vi "Saving to Disk.vi"() -> ()   [LabVIEW 2011]
uses:
  <vilib>/Heliosphere Research LLC/Advanced Plotting Toolkit/Advanced Plotting Toolkit.lvlib
  <vilib>/Utility/sysdir.llb/System Directory Type.ctl
  <vilib>/Heliosphere Research LLC/Advanced Plotting Toolkit/properties/Line_Style.ctl
  <vilib>/Heliosphere Research LLC/Advanced Plotting Toolkit/typedefs/PlotColor.ctl
  <vilib>/Heliosphere Research LLC/Advanced Plotting Toolkit/properties/Line.ctl
  <vilib>/Heliosphere Research LLC/Advanced Plotting Toolkit/properties/Display.ctl
  <vilib>/Heliosphere Research LLC/Advanced Plotting Toolkit/api_plotting/ContourProperties.ctl
  <vilib>/Heliosphere Research LLC/Advanced Plotting Toolkit/api_plotting/Contour_Automatic.vi
panel:
  out "Error from Save":errorcluster
  in  "File Name (on your Desktop)":string="SavedPlot.pdf"
  out "Contour Plot":picture
  # "Saving to Disk"
  # "This VI demonstrates how to save a plot to disk.\n\nPDF save format will preserve lines, arrows, text, etc., as \nresolution-independent vector art.  Raster formats like PNG\nuse advanced anti-aliasing for high quality.\n\nThe format is automatically determined from the file extension\n(case-insensitive).  You can also manually force a particular\nformat using the File Format terminal to Save.vi; for example,\nwhen saving to a file name with no extension.\n\nTip: use Size.vi just before Save.vi if you want to change the\nsize of the plot.\n\n\nFormats:\n\nPDF (.pdf)\nPNG (.png)\nBMP (.bmp)\nTIFF (.tif, .tiff)\nJPEG (.jpg, .jpeg)\nGIF (.gif)"
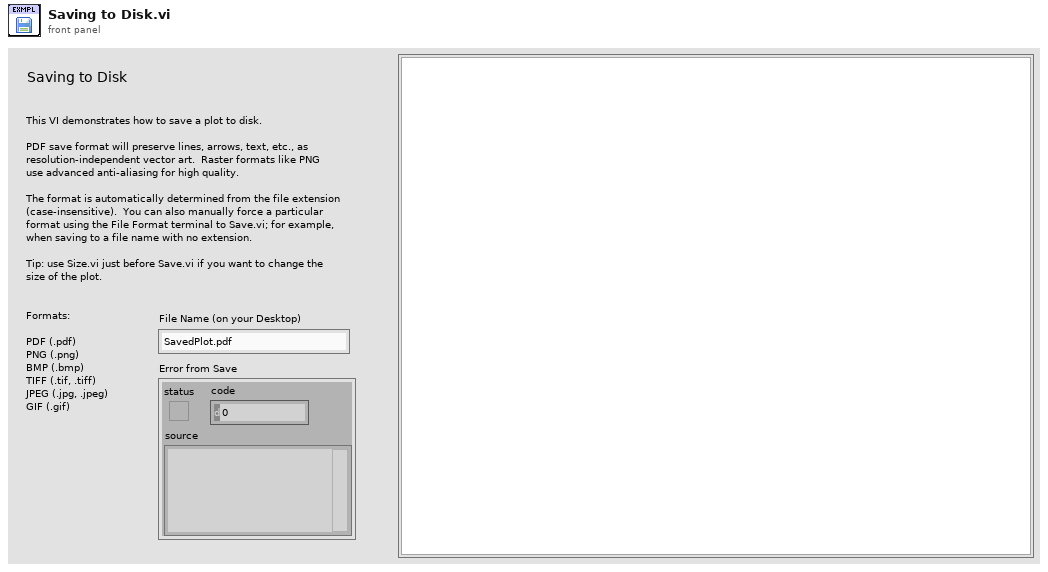
[diagram p1: front panel]
types:
  T1 = typedef "Advanced Plotting Toolkit.lvlib/ContourProperties.ctl" = cluster{"Label Contours":bool, "Line":T2, "Display":T5}
  T2 = typedef "Advanced Plotting Toolkit.lvlib/Line.ctl" = cluster{"Style":T3, "Color":T4, "Width":sgl}
  T3 = typedef "Advanced Plotting Toolkit.lvlib/Line_Style.ctl" = enum16{"Automatic", "Solid", "Dashed", "Dotted", "Dash-dot", "Invisible"}
  T4 = typedef "Advanced Plotting Toolkit.lvlib/PlotColor.ctl" = u32
  T5 = typedef "Advanced Plotting Toolkit.lvlib/Display.ctl" = cluster{"Alpha":dbl, "Z Order":dbl}
  T6 = typedef "System Directory Type.ctl" = i32
  T7 = typedef "Advanced Plotting Toolkit.lvlib/PlotID.ctl" = i32
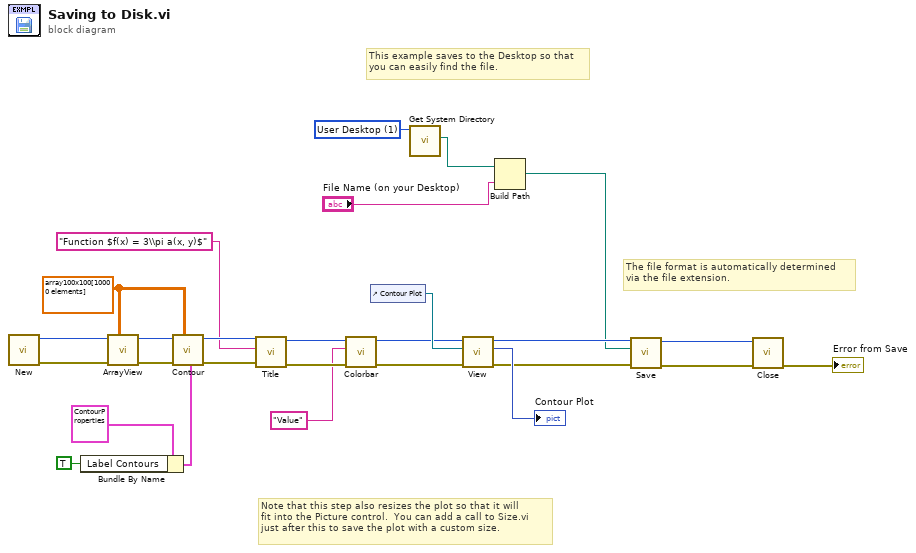
[diagram p0: block diagram]
diagram:
  w17 = T6 1 items=["User Home"=0, "User Desktop"=1, "User Documents"=2, "User Application Data"=3, "User Preferences"=4, "User Temporary"=5, "Public Documents"=6, "Public Application Data"=7, "Public Preferences"=8, "Public Cache"=13, "System Core Libraries"=9, "System Installed Libraries"=10, "Application Files"=11, "Boot Volume Root"=12] ("system directory type")
  w23 = sgl[][] array100x100[10000 elements] ("Array")
  # "Note that this step also resizes the plot so that it will\nfit into the Picture control.  You can add a call to Size.vi\njust after this to save the plot with a custom size."
  # "The file format is automatically determined\nvia the file extension."
  # "This example saves to the Desktop so that\nyou can easily find the file."
  n1 = call <vilib>:"New.vi"() -> ("error out"=w22:errorcluster, "Plot ID"=w25:T7)  [unwired: 10 in]
  n2 = Bundle By Name(cluster=T1 {"Label Contours"=FALSE, "Line"={"Style"=enum."Automatic", "Color"=2147483647, "Width"=nan}, "Display"={"Alpha"=nan, "Z Order"=nan}} ("Contour Properties"), "Label Contours"=TRUE) -> (w9:T1)
  n3 = call <vilib>:"ArrayView.vi"("Data"=w23, "error in (no error)"=w22, "Plot ID"=w25) -> ("error out"=w21:errorcluster, "Plot ID Out"=w24:T7)  [unwired: 7 in]
  n4 = call-poly <vilib>:"Contour.vi"("Properties"=w9, "Z Data"=w23, "error in (no error)"=w21, "Plot ID"=w24) -> ("error out"=w12:errorcluster, "Plot ID Out"=w13:T7)  [unwired: 6 in]
  n5 = call <vilib>:"Title.vi"("error in (no error)"=w12, "Title"="Function $f(x) = 3\\pi a(x, y)$", "Plot ID"=w13) -> ("error out"=w5:errorcluster, "Plot ID out"=w7:T7)  [unwired: 7 in]
  n6 = call <vilib>:"Colorbar.vi"("error in (no error)"=w5, "Label"="Value", "Plot ID"=w7) -> ("error out"=w4:errorcluster, "Plot ID Out"=w6:T7)  [unwired: 7 in]
  n7 = control-ref of="Contour Plot"() -> (w27:refnum<vi>)
  n8 = call <vilib>:"Get System Directory.vi"("system directory type"=w17) -> ("system directory"=w16:path)  [unwired: 10 in]
  n9 = call <vilib>:"View.vi"("error in (no error)"=w4, "Ref for Sizing"=w27, "Plot ID"=w6) -> ("error out"=w19:errorcluster, "Picture"=→"Contour Plot":picture, "Plot ID Out"=w20:T7)  [unwired: 6 in]
  n10 = Build Path(base path=w16, name or relative path="File Name (on your Desktop)") -> (appended path=w14:path)
  n11 = call <vilib>:"Save.vi"("error in (no error)"=w19, "Path"=w14, "Plot ID In"=w20) -> ("error out"=w2:errorcluster, "Plot ID Out"=w18:T7)  [unwired: 7 in]
  n12 = call <vilib>:"Close.vi"("error in (no error)"=w2, "Plot ID"=w18) -> ("error out"=→"Error from Save":errorcluster)  [unwired: 9 in]
